vi "move item between listboxes.vi"(8 "error in":errorcluster, 10 "target":refnum<vi>, 11 "source":refnum<vi>) -> (0 "error out":errorcluster, 2 "new target":string[](array[string]), 3 "new source":string[](array[string]))   [LabVIEW 2013, in "TagBusConfigurablePluginDecideFeatures.lvclass"]
uses:
  TagBusConfigurablePluginDecideFeatures.lvclass
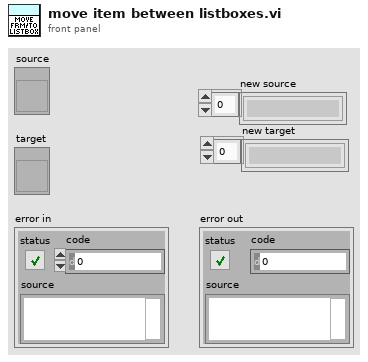
[diagram p1: front panel]
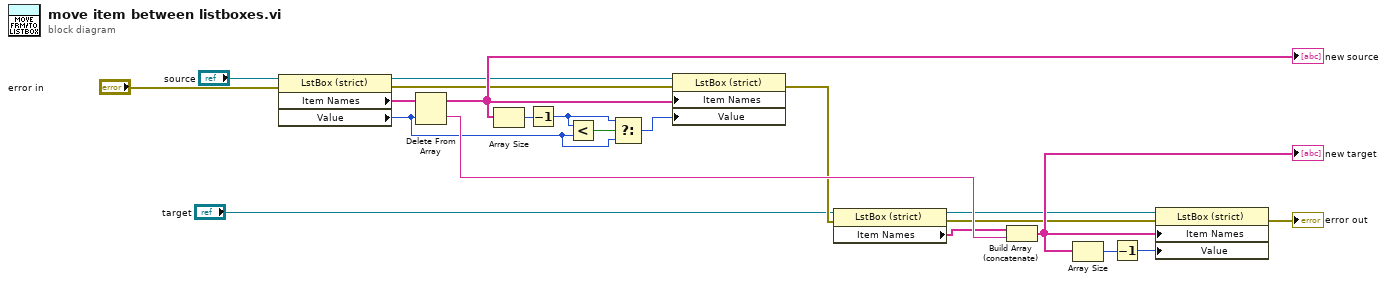
[diagram p0: block diagram]
diagram:
  n1 = property class="LstBox (strict)"(reference="source", error in="error in") -> (reference out=w3:refnum<vi>, error out=w2:errorcluster, "Item Names"=w1:string[], "Value"=w7:i32)
  n2 = Delete From Array(array=w1, index=w7) -> (deleted portion=w18:string, array with subset deleted=w4:string[])  [unwired: 1 in]
  "new source" <- w4
  n3 = Array Size(array=w4) -> (size(s)=w5:i32)
  n4 = Decrement(x=w5) -> (x-1=w8:i32)
  n5 = Less?(x=w8, y=w7) -> (x < y?=w6:bool)
  n6 = Select(t=w8, s=w6, f=w7) -> (s? t:f=w9:i32)
  n7 = property class="LstBox (strict)"(reference=w3, error in=w2, "Item Names"=w4, "Value"=w9) -> (error out=w14:errorcluster)  [unwired: 1 out]
  n8 = property class="LstBox (strict)"(reference="target", error in=w14) -> (reference out=w11:refnum<vi>, error out=w12:errorcluster, "Item Names"=w17:string[])
  n9 = Build Array (concatenate)(w17, w18) -> (w19:string[])
  "new target" <- w19
  n10 = Array Size(array=w19) -> (size(s)=w21:i32)
  n11 = Decrement(x=w21) -> (x-1=w20:i32)
  n12 = property class="LstBox (strict)"(reference=w11, error in=w12, "Item Names"=w19, "Value"=w20) -> (error out=→"error out":errorcluster)  [unwired: 1 out]
